vi "I2C_MASTER_WRITE.vi"(1 "error in (no error)":errorcluster, 2 "Latch":bool, 3 "Mode":T1) -> (0 "error out":errorcluster)   [LabVIEW 2018]
uses:
  I2C_MASTER_WRITE.ctl
  <vilib>/Studica/Studica Toolkit/Background/I2C Channel.ctl
panel:
  out "Data To Write":u8[](array[numeric])
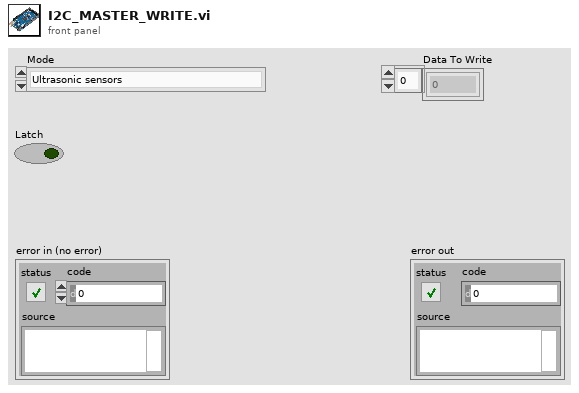
[diagram p1: front panel]
types:
  T1 = typedef "I2C_MASTER_WRITE.ctl" = enum16{"Ultrasonic sensors", "Stepper origin", "zStepper 13.3k", "zStepper 13k", "zStepper 12k", "zStepper 11k", "zStepper 10k", "zStepper 9k", "zStepper 8k", "zStepper 7k", "zStepper 6k", "zStepper 5k", "zStepper 4k", "zStepper 3k", "zStepper 2k", "zStepper 1k", "zStepper 900", "zStepper 800", "zStepper 700", "zStepper 600", "zStepper 500", "zStepper 400", "zStepper 300", "zStepper 200", "zStepper 100", "zStepper 0", "yStepper 4.7k", "yStepper 4.6k", "yStepper 4.5k", "yStepper 4.4k", "yStepper 4.3k", "yStepper 4.2k", "yStepper 4.1k", "yStepper 4k", "yStepper 3.9k", "yStepper 3.8k", "yStepper 3.7k", "yStepper 3.6k", "yStepper 3.5k", "yStepper 3.4k", "yStepper 3.3k", "yStepper 3.2k", "yStepper 3.1k", "yStepper 3k", "yStepper 2.9k", "yStepper 2.8k", "yStepper 2.7k", "yStepper 2.6k", "yStepper 2.5k", "yStepper 2.4k", "yStepper 2.3k", "yStepper 2.2k", "yStepper 2.1k", "yStepper 2k", "yStepper 1.9k", "yStepper 1.8k", "yStepper 1.7k", "yStepper 1.6k", "yStepper 1.5k", "yStepper 1.4k", "yStepper 1.3k", "yStepper 1.2k", "yStepper 1.1k", "yStepper 1k", "yStepper 900", "yStepper 800", "yStepper 700", "ySteppre 600", "yStepper 500", "yStepper 400", "yStepper 300", "yStepper 200", "yStepper 100", "yStepper 0", "Open claw", "Close claw", "Last State", "Manual y stepper"}
  T2 = typedef "I2C Channel.ctl" = enum16{"Not Connected", "A", "B"}
  T3 = cluster{"I2C Channel":T2, "FPGA VI Reference Out":refnum<k20>}
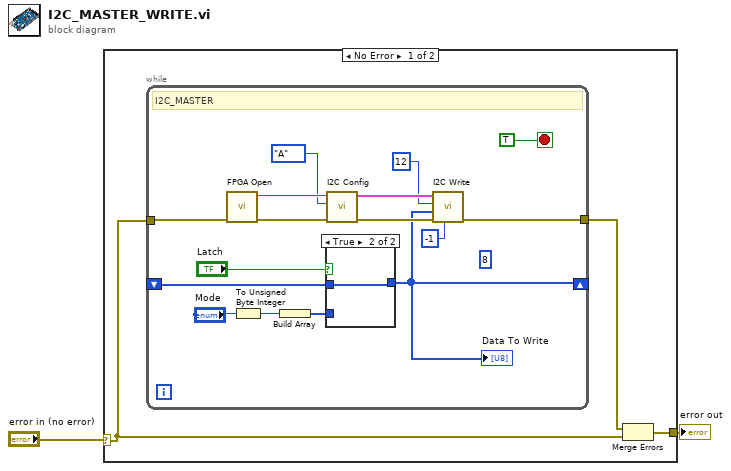
[diagram p0: block diagram]
diagram:
  n1 = case shown="No Error" "error in (no error)" {
    selector: "error in (no error)" -> [w4 w24]
    tunnel: [w5 w24] -> w1
    frame No Error {
      n2 = while {
        tunnel: w4 -> [w13]
        shift-right: [w9] -> _
        shift-left: _ -> [w7]
        tunnel: [w6] -> w3
        stop <- TRUE ("stop") stop-if-true
        (unwired) u32 8 ("Bytes to Read")
        # "I2C_MASTER"
        n3 = call <vilib>:"FPGA Open.vi"("error in (no error)"=w13) -> ("error out"=w19:errorcluster, "FPGA Reference Out"=w20:refnum<k20>)  [unwired: 9 in]
        n4 = To Unsigned Byte Integer(number="Mode") -> (unsigned 8bit integer=w11:u8)
        n5 = Build Array(w11) -> (w10:u8[])
        n6 = case shown="True" "Latch" {
          tunnel: w10 -> [w22 _]
          tunnel: [w22 w23] -> w9
          tunnel: w7 -> [_ w23]
          frame False {
          }
          frame True {
          }
        }
        "Data To Write" <- w9
        n7 = call <vilib>:"I2C Config.vi"("error in (no error)"=w19, "I2C Channel"=I2C_Channel."A", "FPGA Reference"=w20) -> ("error out"=w16:errorcluster, "I2C Ref Out"=w17:T3)  [unwired: 7 in]
        n8 = call <vilib>:"I2C Write.vi"("Timeout ms (1000)"=-1, "error in (no error)"=w16, "Data to Write"=w9, "Slave Address (7-bit)"=u8 12, "I2C Ref In"=w17) -> ("error out"=w6:errorcluster)  [unwired: 5 in, 1 out]
      }
      n9 = Merge Errors(w3, w4) -> (w5:errorcluster)
    }
    frame Error {
    }
  }
  "error out" <- w1
